vi "CutAndBinImages.vi"(10 "Intensity Graph":i32[][](graph)) -> (1 "Background Image":i32[][](graph), 2 "Atom Image":i32[][](graph))   [LabVIEW 2015]
uses:
  Controls/PixelFly/Acquisition Settings.ctl
panel:
  out "Acquitsition Settings":T1
  out "size(s) 2":i32[](array[numeric])
  out "size(s)":i32[](array[numeric])
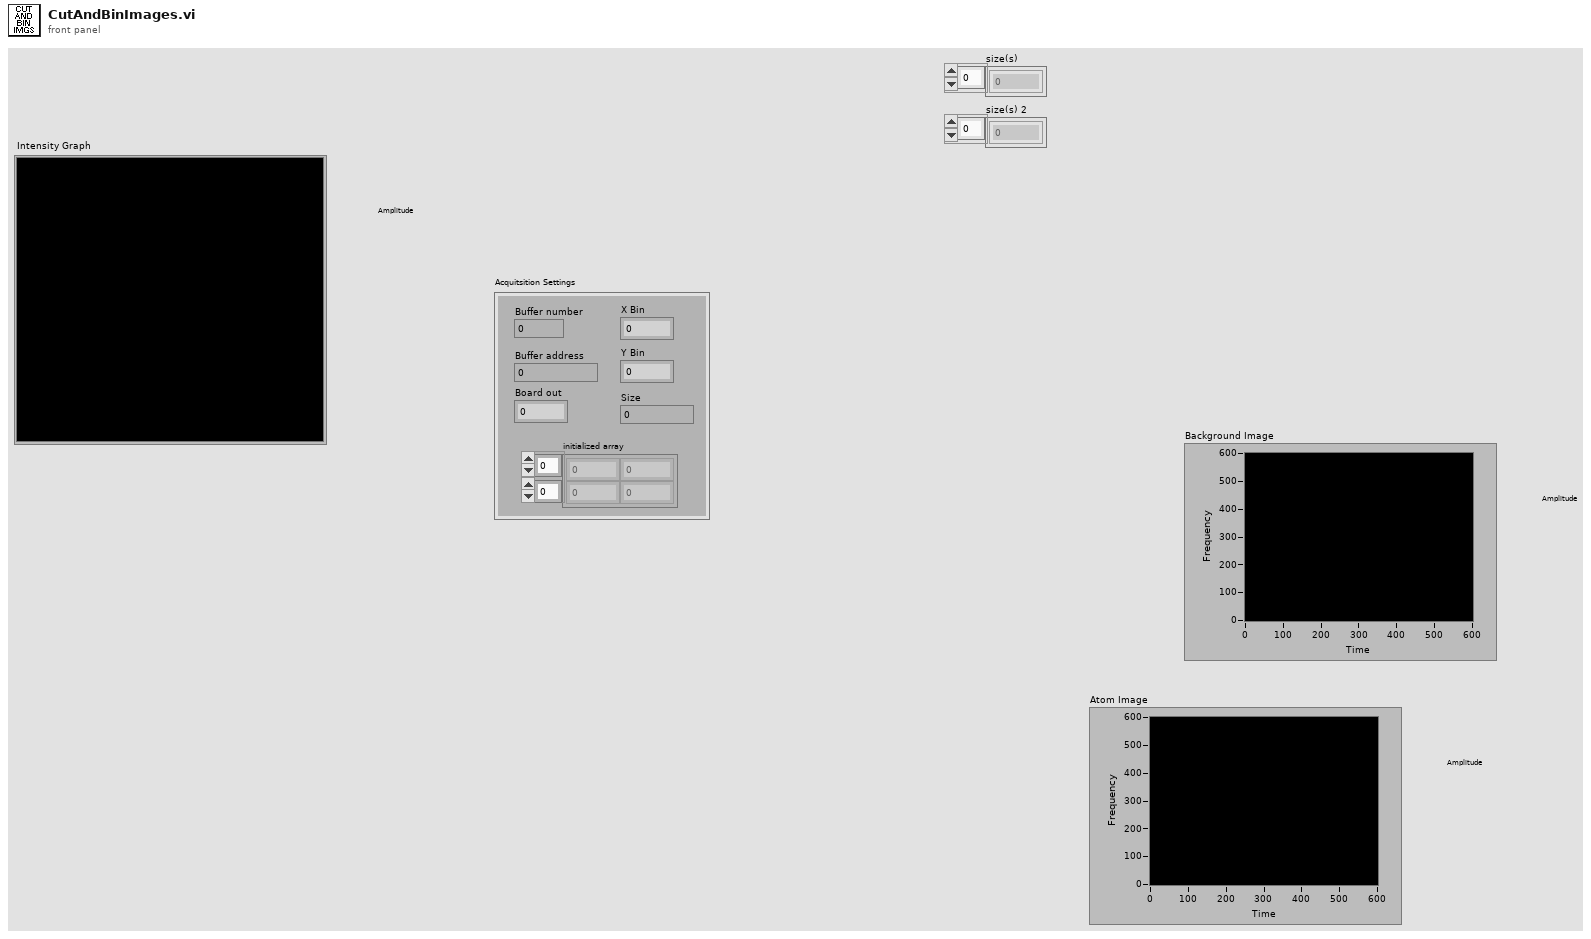
[diagram p1: front panel]
types:
  T1 = typedef "Acquisition Settings.ctl" = cluster{"Buffer number":i32, "Buffer address":i32, "Size":i32, "initialized array":u8[][], "X Bin":i32, "Y Bin":i32, "Board out":dbl}
  T2 = typedef "camera_controls.ctl" = cluster{"Acquisition Mode":T3, "Trigger Mode":T4, "Frame \nTransfer":bool, "Exposure Time (s)":sgl, "Accumulation Cycle Time (s)":sgl, "# Accumulations":i32, "# Kinetics":i32, "Kinetic Cycle Time (s)":sgl, "Horizontal Bin Size":i32, "Vertical Bin Size":i32}
  T3 = typedef "AcquisitionMode_mode typedef.ctl" = enum16{"Reserved (0)", "Single Scan", "Accumulate", "Kinetics", "Fast Kinetics", "Run Till Abort", "Reserved (6)", "Reserved (7)", "Reserved (8)", "Time Delayed Integration"}
  T4 = typedef "TriggerMode_mode typedef.ctl" = enum16{"Internal", "External", "N/A (2)", "N/A (3)", "N/A (4)", "N/A (5)", "External Start", "External Exposure (Bulb)", "N/A (8)", "External FVB EM", "Software", "N/A (11)", "External Charge Shifting"}
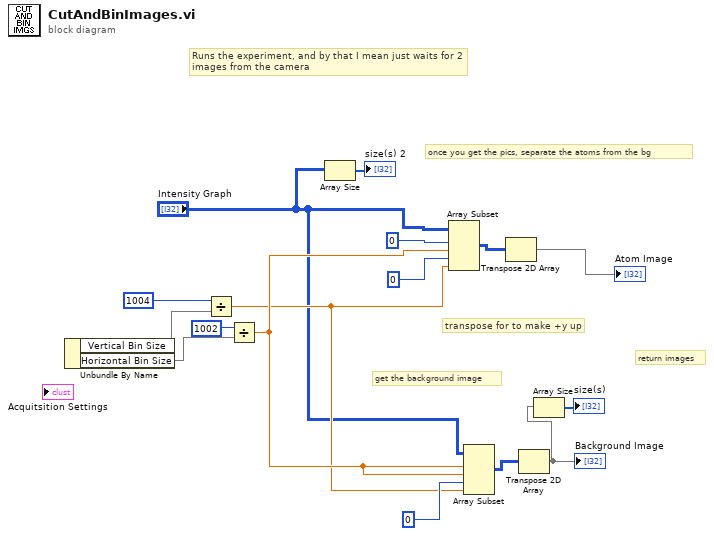
[diagram p0: block diagram]
diagram:
  # "return images"
  # "transpose for to make +y up"
  # "get the background image"
  # "once you get the pics, separate the atoms from the bg"
  # "Runs the experiment, and by that I mean just waits for 2\nimages from the camera"
  n1 = Unbundle By Name() -> (w12:T2, "Vertical Bin Size"=w10, "Horizontal Bin Size"=w8)
  n2 = Divide(x=1004 ("length"), y=w10) -> (x/y=w2:dbl)
  n3 = Divide(x=1002 ("length"), y=w8) -> (x/y=w3:dbl)
  n4 = Array Size(array="Intensity Graph") -> (size(s)=→"size(s) 2":i32[])
  n5 = Array Subset(array="Intensity Graph", index (row)=0, length (row)=w3, index (col)=0 ("index"), length (col)=w2) -> (w14:i32[][])
  n6 = Array Subset(array="Intensity Graph", index (row)=w3, length (row)=w3, index (col)=0 ("index"), length (col)=w2) -> (w7:i32[][])
  n7 = Transpose 2D Array(2D array=w14) -> (transposed array=→"Atom Image":i32[][])
  n8 = Transpose 2D Array(2D array=w7) -> (transposed array=w4:i32[][])
  "Background Image" <- w4
  n9 = Array Size(array=w4) -> (size(s)=→"size(s)":i32[])
